vi "Angle to Pot.Voltage_subVI.vi"(11 "Pull-back angle (°)":dbl) -> (3 "Potentiometer V (0-5)":dbl)   [LabVIEW 2017]
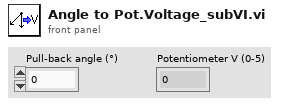
[diagram p1: front panel]
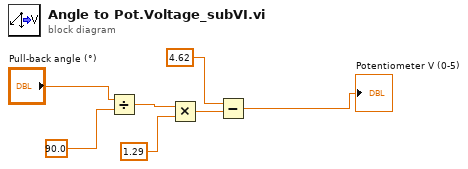
[diagram p0: block diagram]
diagram:
  n1 = Divide(x="Pull-back angle (°)", y=90.0) -> (x/y=w3:dbl)
  n2 = Multiply(x=w3, y=1.29) -> (x*y=w5:dbl)
  n3 = Subtract(x=4.62, y=w5) -> (x-y=→"Potentiometer V (0-5)":dbl)
